vi "Write to cRIO_SIL.vi"(8 "error in (no error)":errorcluster, 11 "Vessel in":refnum<class "Vessel.lvclass">) -> (0 "error out":errorcluster, 2 "telebuf":u8[](array[numeric]), 3 "Vessel out":refnum<class "Vessel.lvclass">)   [LabVIEW 2014, in "Vessel.lvclass"]
uses:
  Vessel.lvclass
  Vessel.lvclass/Vessel.ctl
  Supervisor/Supervisor.lvclass
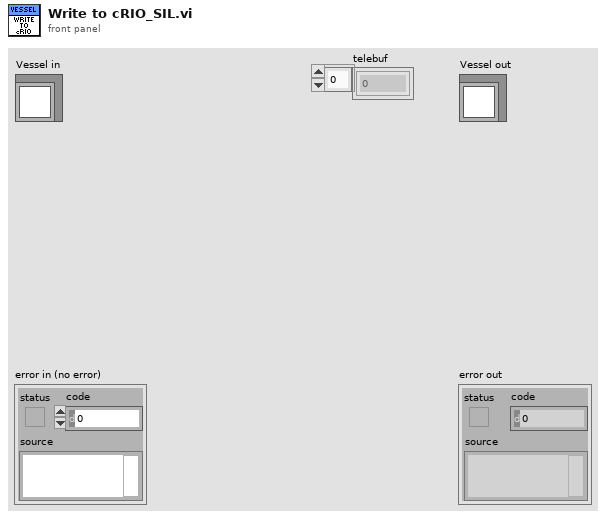
[diagram p1: front panel]
types:
  T1 = cluster{"Measured":cluster{"Eta":dbl[], "Nu":dbl[], "Eta Dot":dbl[], "Nu Dot":dbl[]}, "Estimated":cluster{"Eta":dbl[], "Nu":dbl[], "Eta Dot":dbl[], "Nu Dot":dbl[]}, "Desired":cluster{"Eta":dbl[], "Nu":dbl[], "Eta Dot":dbl[], "Nu Dot":dbl[]}, "Previous Desired":cluster{"Eta":dbl[], "Nu":dbl[], "Eta Dot":dbl[], "Nu Dot":dbl[]}, "tau":dbl[], "Altitude":cluster{"Measured":dbl, "Estimated":dbl, "Desired":dbl, "Previous Desired":dbl, "Approximated":dbl, "grad F":dbl[]}, "rpm":dbl[], "Attitude":cluster{"Theta Measured":dbl[], "Theta Estimated":dbl[], "Omega Measured":dbl[], "Omega Estimated":dbl[], "Gyro Bias":dbl[]}}
  T2 = cluster{"Set Origin":bool, "New WP":bool, "Types of Change":enum16{"Current NED", "Change NED"}, "Make Change":bool, "Optimal Heading":bool, "New SetPoint":cluster{"North":dbl, "East":dbl, "Depth":dbl, "Heading":dbl}, "Update Reference":cluster{"Mode Change":bool, "Current Position":dbl[]}, "Go":bool, "Go heading":bool}
  T3 = cluster{"Power Switch":bool, "Upper Arm Up":bool, "Upper Arm Down":bool, "Lower Arm Up":bool, "Lower Arm Down":bool, "Arm Left":bool, "Arm Right":bool, "Claw Open":bool, "Claw Close":bool, "Rotate Clockwise":bool, "Rotate Counterclockwise":bool}
  T4 = cluster{"Light 1":bool, "Light 2":bool, "Light 3":bool, "Light 4":bool, "HMI 1":bool, "HMI 2":bool, "Light Intensity 1":i32, "Light Intensity 2":i32, "Light Intensity 3":i8}
  T5 = cluster{"Eta":dbl[], "Nu":dbl[], "Eta Dot":dbl[], "Nu Dot":dbl[]}
  T6 = cluster{"Cam. No.":i32, "Cam Up":bool, "Cam Down":bool, "Cam Left":bool, "Cam Right":bool, "Zoom In":bool, "Zoom Out":bool, "Zoom In 2":bool, "Zoom Out 2":bool}
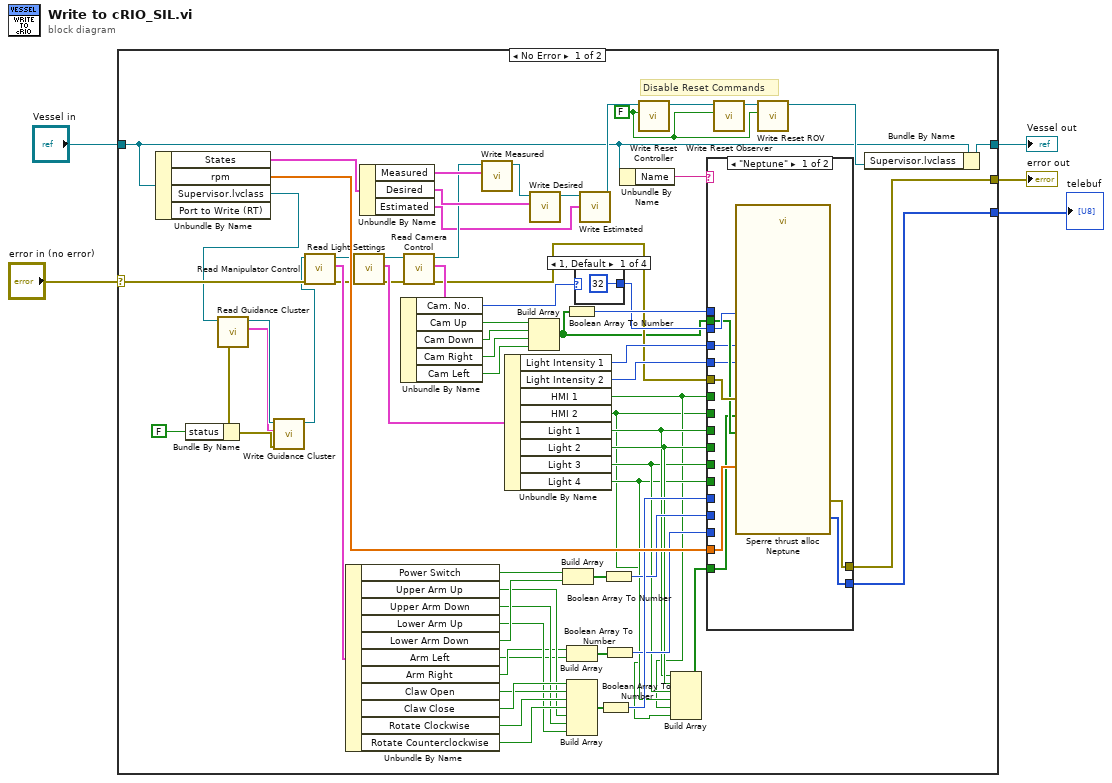
[diagram p0: block diagram]
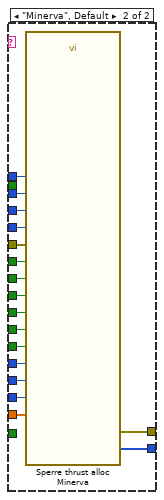
[diagram p2: hidden frame]
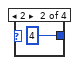
[diagram p3: hidden frame]
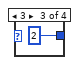
[diagram p4: hidden frame]
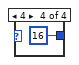
[diagram p5: hidden frame]
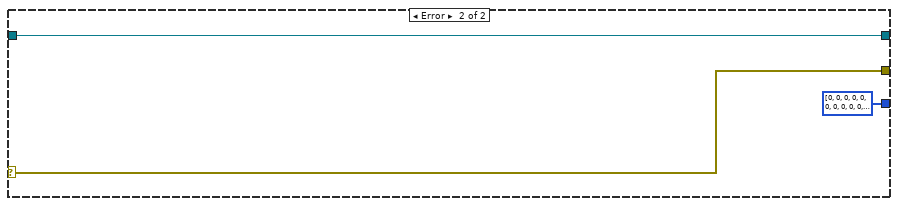
[diagram p6: hidden frame]
diagram:
  n1 = case shown="No Error" "error in (no error)" {
    selector: "error in (no error)" -> [w41 w106]
    tunnel: [w37 w106] -> w4
    tunnel: [w30 w105] -> w2
    tunnel: "Vessel in" -> [w18 w105]
    tunnel: [w36 u8[] [0, 0, 0, 0, 0, 0, 0, 0, 0, 0, 0, 0, 0, 0, 0, 0, 0, 0] ("telebuf")] -> w1
    frame No Error {
      w19 = FALSE ("Reset Controller")
      # "Disable Reset Commands"
      n2 = Unbundle By Name(w18) -> ("States"=w35:T1, "rpm"=w73:dbl[], "Supervisor.lvclass"=w26:refnum<class "Supervisor.lvclass">)  [unwired: 1 out]
      n3 = call-dynamic "Read Guidance Cluster.vi"("Supervisor in"=w26) -> ("error out"=w24:errorcluster, "Guidance Cluster"=w6:T2, "Supervisor out"=w27:refnum<class "Supervisor.lvclass">)  [unwired: 8 in]
      n4 = Bundle By Name(cluster=w24, "status"=FALSE ("Set Origin")) -> (w8:errorcluster)
      n5 = call-dynamic "Write Guidance Cluster.vi"("error in (no error)"=w8, "Guidance Cluster"=w6, "Supervisor in"=w27) -> ("Supervisor out"=w25:refnum<class "Supervisor.lvclass">)  [unwired: 7 in, 1 out]
      n6 = call-dynamic "Read Manipulator Control.vi"("error in (no error)"=w41, "Supervisor in"=w25) -> ("error out"=w40:errorcluster, "Manipulator Control"=w61:T3, "Supervisor out"=w43:refnum<class "Supervisor.lvclass">)  [unwired: 7 in]
      n7 = Unbundle By Name(w61) -> ("Power Switch"=w60:bool, "Upper Arm Up"=w54:bool, "Upper Arm Down"=w53:bool, "Lower Arm Up"=w52:bool, "Lower Arm Down"=w59:bool, "Arm Left"=w50:bool, "Arm Right"=w51:bool, "Claw Open"=w57:bool, "Claw Close"=w58:bool, "Rotate Clockwise"=w56:bool, "Rotate Counterclockwise"=w55:bool)
      n8 = call-dynamic "Read Light Settings.vi"("error in (no error)"=w40, "Supervisor in"=w43) -> ("error out"=w39:errorcluster, "Light Settings"=w62:T4, "Supervisor out"=w42:refnum<class "Supervisor.lvclass">)  [unwired: 7 in]
      n9 = Unbundle By Name(w35) -> ("Measured"=w34:T5, "Desired"=w33:T5, "Estimated"=w28:T5)
      n10 = call-dynamic "Read Camera Control.vi"("error in (no error)"=w39, "Supervisor in"=w42) -> ("error out"=w38:errorcluster, "Camera Control"=w70:T6, "Supervisor out"=w32:refnum<class "Supervisor.lvclass">)  [unwired: 7 in]
      n11 = Unbundle By Name(w70) -> ("Cam. No."=w64:i32, "Cam Up"=w69:bool, "Cam Down"=w68:bool, "Cam Right"=w67:bool, "Cam Left"=w66:bool)
      n12 = call-dynamic "Write Measured.vi"("Measured"=w34, "Supervisor in"=w32) -> ("Supervisor out"=w31:refnum<class "Supervisor.lvclass">)  [unwired: 8 in, 1 out]
      n13 = Unbundle By Name(w62) -> ("Light Intensity 1"=w72:i32, "Light Intensity 2"=w71:i32, "HMI 1"=w11:bool, "HMI 2"=w10:bool, "Light 1"=w14:bool, "Light 2"=w15:bool, "Light 3"=w13:bool, "Light 4"=w12:bool)
      n14 = Build Array(w69, w68, w67, w66) -> (w16:bool[])
      n15 = call-dynamic "Write Desired.vi"("Desired"=w33, "Supervisor in"=w31) -> ("Supervisor out"=w29:refnum<class "Supervisor.lvclass">)  [unwired: 8 in, 1 out]
      n16 = Build Array(w60, w59) -> (w49:bool[])
      n17 = Boolean Array To Number(Boolean array=w16) -> (number=w65:u32)
      n18 = Build Array(w51, w50) -> (w47:bool[])
      n19 = Build Array(w58, w57, w56, w55, w54, w53, w52) -> (w48:bool[])
      n20 = case shown="1, Default" w64 {
        tunnel: [32 4 2 16] -> w63
        frame 1, Default {
        }
        frame 2 {
        }
        frame 3 {
        }
        frame 4 {
        }
      }
      n21 = call-dynamic "Write Estimated.vi"("Estimated"=w28, "Supervisor in"=w29) -> ("Supervisor out"=w22:refnum<class "Supervisor.lvclass">)  [unwired: 8 in, 1 out]
      n22 = Boolean Array To Number(Boolean array=w48) -> (number=w46:u32)
      n23 = Boolean Array To Number(Boolean array=w49) -> (number=w45:u32)
      n24 = Boolean Array To Number(Boolean array=w47) -> (number=w44:u32)
      n25 = Unbundle By Name(w18) -> ("Name"=w17:string)
      n26 = call-dynamic "Write Reset Controller.vi"("Reset Controller"=w19, "Supervisor in"=w22) -> ("Supervisor out"=w23:refnum<class "Supervisor.lvclass">)  [unwired: 8 in, 1 out]
      n27 = Build Array(w14, w15, w13, w12, w11, w10) -> (w9:bool[])
      n28 = case shown="\"Neptune\"" w17 {
        tunnel: w73 -> [w81 w99]
        tunnel: w11 -> [_ w98]
        tunnel: w10 -> [_ w97]
        tunnel: w14 -> [_ w96]
        tunnel: w15 -> [_ w95]
        tunnel: w13 -> [_ w94]
        tunnel: w12 -> [_ w93]
        tunnel: w72 -> [w75 w92]
        tunnel: w71 -> [w74 w91]
        tunnel: w65 -> [_ w90]
        tunnel: w63 -> [w78 w89]
        tunnel: w46 -> [_ w88]
        tunnel: w45 -> [_ w87]
        tunnel: w44 -> [_ w86]
        tunnel: w38 -> [w82 w85]
        tunnel: [w79 w84] -> w37
        tunnel: [w80 w83] -> w36
        tunnel: w16 -> [w77 _]
        tunnel: w9 -> [w76 _]
        frame "Neptune" {
          n29 = call "Sperre thrust alloc Neptune.vi"("Thruster rpms"=w81, "pan tilt"=w77, "Lights/HMI"=w76, "error in"=w82, "dim 1"=w75, "dim 2"=w74, "cam no"=w78) -> ("telebuf out"=w80:u8[], "error IO"=w79:errorcluster)  [unwired: 11 in]
        }
        frame "Minerva", Default {
          n30 = call "Sperre thrust alloc Minerva.vi"("Thruster rpms"=w99, "manip14"=w88, "manip15"=w87, "manip16"=w86, "error in"=w85, "dim 1+2"=w92, "Light 1"=w96, "dim 3+4"=w91, "Light 2"=w95, "digital2"=w90, "Light 3"=w94, "camera"=w89, "Light 4"=w93, "HMI 1"=w98, "HMI 2"=w97) -> ("telebuf"=w83:u8[], "error IO"=w84:errorcluster)  [unwired: 3 in]
        }
      }
      n31 = call-dynamic "Write Reset Observer.vi"("Reset Observer"=w19, "Supervisor in"=w23) -> ("Supervisor out"=w21:refnum<class "Supervisor.lvclass">)  [unwired: 8 in, 1 out]
      n32 = call-dynamic "Write Reset ROV.vi"("Reset ROV"=w19, "Supervisor in"=w21) -> ("Supervisor out"=w20:refnum<class "Supervisor.lvclass">)  [unwired: 8 in, 1 out]
      n33 = Bundle By Name(cluster=w18, "Supervisor.lvclass"=w20) -> (w30:refnum<class "Vessel.lvclass">)
    }
    frame Error {
    }
  }
  "error out" <- w4
  "Vessel out" <- w2
  "telebuf" <- w1
